vi "SDKSID4_Grab Image.vi"(7 "error in (no error)":errorcluster, 10 "SDKSID4 session In":T1) -> (0 "error out":errorcluster, 2 "Image":i16[][](array[numeric]), 3 "SDKSID4 session Out":T1)   [LabVIEW 2013]
doc: "This VI grabs an image from the camera and output it as a signed short integer (I16) array of numbers. You need to call Start Live Mode before calling this VI to be able to grab any image.\nNote : in the image, X and Y are inverted."
uses:
  Refnum SDKSID4 session.ctl
  SDKSID4_ImageCameraSize.ctl
  SID4_SDK.dll
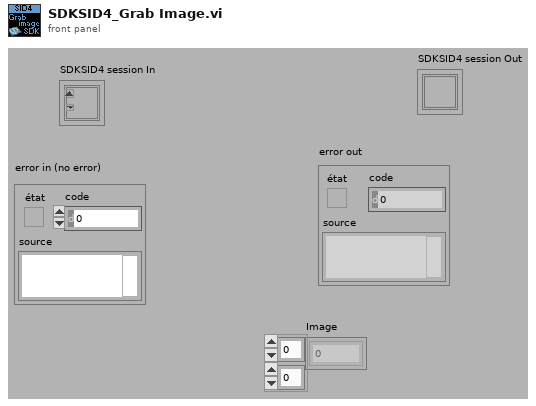
[diagram p1: front panel]
types:
  T1 = typedef "Refnum SDKSID4 session.ctl" = refnum<k1>
  T2 = typedef "SDKSID4_ImageCameraSize.ctl" = cluster{"nRow":i32, "nCol":i32}
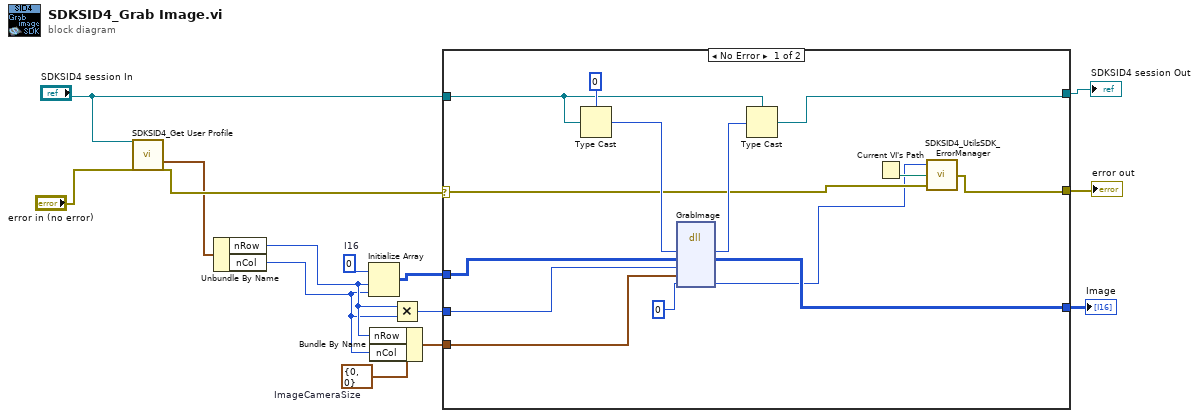
[diagram p0: block diagram]
diagram:
  w9 = T2 {"nRow"=0, "nCol"=0}  # ImageCameraSize
  w12 = i16 0  # I16
  n1 = call "SDKSID4_Get User Profile.vi"("SDKSID4 session In"="SDKSID4 session In", "error in"="error in (no error)") -> ("ImageCameraSize"=w4:T2, "error out"=w5:errorcluster)  [unwired: 14 in, 10 out]
  n2 = Unbundle By Name(w4) -> ("nRow"=w3:i32, "nCol"=w2:i32)
  n3 = Initialize Array(w12, w3, w2) -> (w11:i16[][])
  n4 = Bundle By Name(cluster=w9, "nRow"=w3, "nCol"=w2) -> (w8:T2)
  n5 = Multiply(x=w3, y=w2) -> (x*y=w7:i32)
  n6 = case shown="No Error" w5 {
    selector: w5 -> [w17 w31]
    tunnel: "SDKSID4 session In" -> [w25 w30]
    tunnel: [w24 w30] -> w14
    tunnel: [w15 w31] -> w10
    tunnel: [w23 w29] -> w13
    tunnel: w11 -> [w22 w29]
    tunnel: w8 -> [w20 _]
    tunnel: w7 -> [w19 _]
    frame No Error {
      n7 = Type Cast(type=u32 0, x=w25) -> (*(type *) &x=w28:u32)
      n8 = dll-call lib="C:/Program Files/SID4_SDK/DLL SDK/BIN/SID4_SDK.dll" fn="GrabImage"("SID4Session"=w28, "ImageI16"=w22, "image_bufSize"=w19, "ImageCameraSize"=w20, "Error"=0) -> ("SID4Session"=w26:u32, "ImageI16"=w23:i16[][], "Error"=w16:i32)  [unwired: 6 in, 2 out]
      n9 = Type Cast(type=w25, x=w26) -> (*(type *) &x=w24:T1)
      n10 = Current VI's Path() -> (path=w18:path)
      n11 = call "SDKSID4_UtilsSDK_ErrorManager.vi"("error IN"=w17, "VI PathFile"=w18, "ErrorCode"=w16) -> ("error OUT"=w15:errorcluster)
    }
    frame Error {
    }
  }
  "error out" <- w10
  "SDKSID4 session Out" <- w14
  "Image" <- w13
